vi "ShoulderEncoderToAngle.vi"(11 "encoderPulses":i32) -> (3 "shoulder angle(deg)":dbl, 5 "Negative":bool)   [LabVIEW 2018]
uses:
  Arm Constants.vi
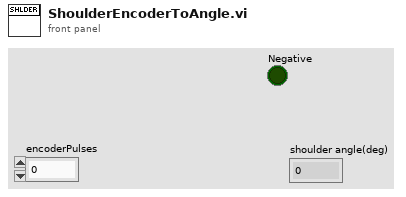
[diagram p1: front panel]
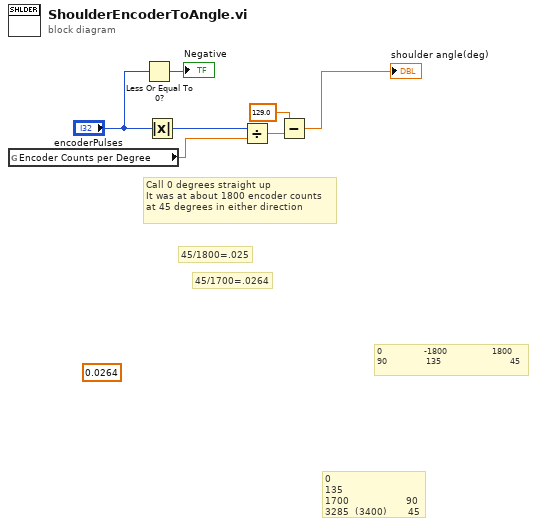
[diagram p0: block diagram]
diagram:
  (unwired) 0.0264 ("y")
  # "45/1700=.0264"
  # "0                         135\n1700                   90\n3285  (3400)       45"
  # "0              -1800               1800\n90             135                       45"
  # "45/1800=.025"
  # "Call 0 degrees straight up\nIt was at about 1800 encoder counts\nat 45 degrees in either direction"
  n1 = global read "Arm Constants.vi" "Encoder Counts per Degree"() -> (w1:dbl)
  n2 = Less Or Equal To 0?(x="encoderPulses") -> (x <= 0?=→"Negative":bool)
  n3 = Absolute Value(x="encoderPulses") -> (abs(x)=w7:i32)
  n4 = Divide(x=w7, y=w1) -> (x/y=w6:dbl)
  n5 = Subtract(x=129.0, y=w6) -> (x-y=→"shoulder angle(deg)":dbl)
